vi "Scrape Matplotlib Color Map Hacking.vi"() -> ()   [LabVIEW 2019]
uses:
  <vilib>/Utility/sysdir.llb/System Directory Type.ctl
panel:
  out "Colormap Map":map{string, u32[]}(c390)
  out "Colormap Names":string[](array[string])
  out "Intensity Graph 2":dbl[][](graph)
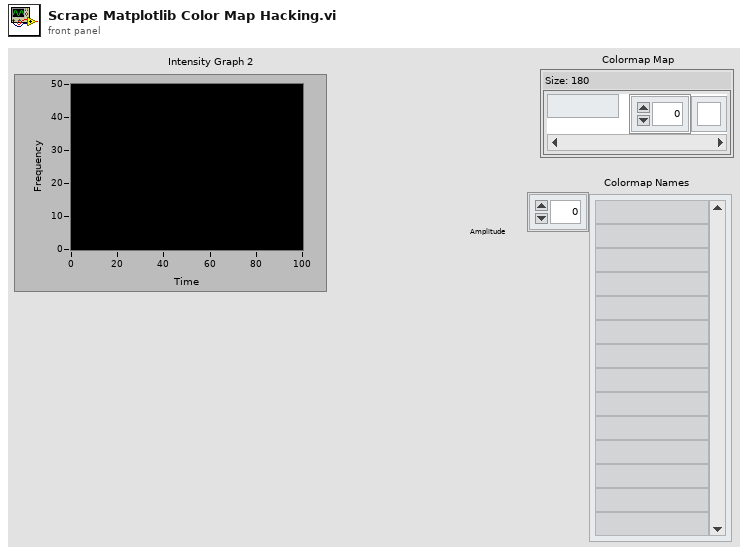
[diagram p1: front panel]
types:
  T1 = enum16{"open", "replace", "create", "open or create", "replace or create", "replace or create with confirmation"}
  T2 = typedef "System Directory Type.ctl" = i32
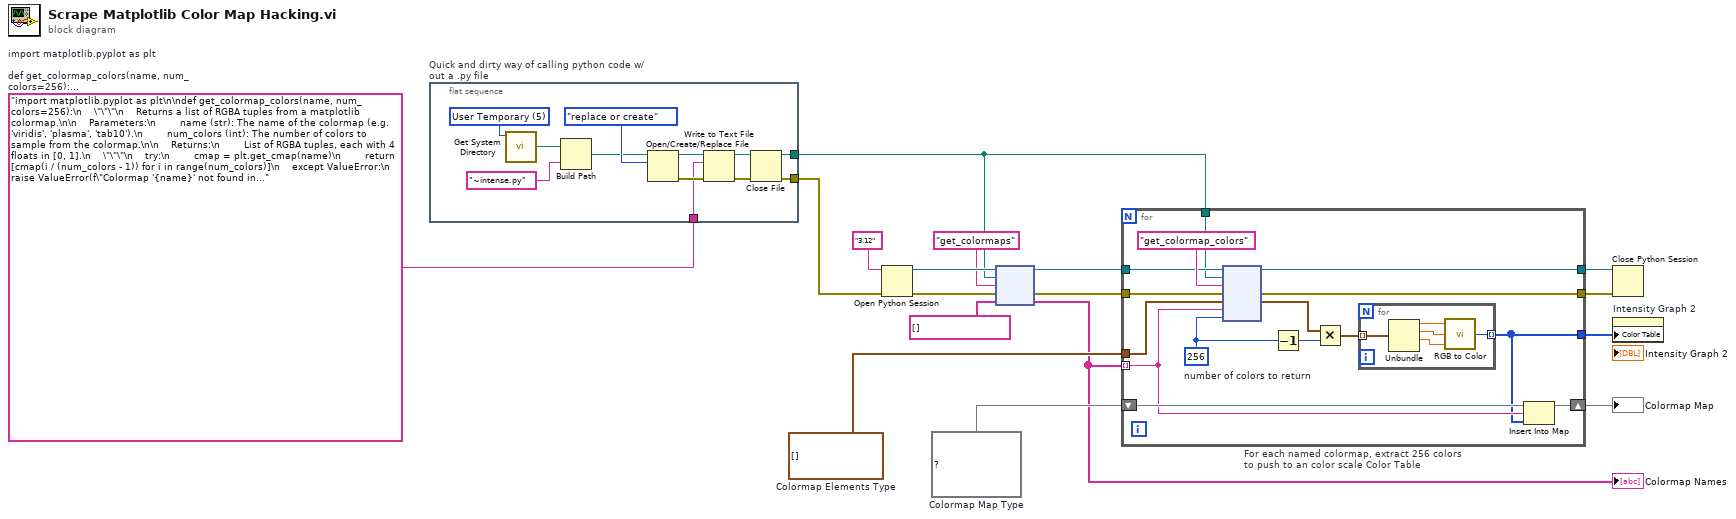
[diagram p0: block diagram]
diagram:
  w2 = cluster{"R":dbl, "G":dbl, "B":dbl, "A":dbl}[] []  # Colormap Elements Type
  w8 = map{string, u32[]} {}  # Colormap Map Type
  w3 = "import matplotlib.pyplot as plt\n\ndef get_colormap_colors(name, num_colors=256):\n    \"\"\"\n    Returns a list of RGBA tuples from a matplotlib colormap.\n\n    Parameters:\n        name (str): The name of the colormap (e.g. 'viridis', 'plasma', 'tab10').\n        num_colors (int): The number of colors to sample from the colormap.\n\n    Returns:\n        List of RGBA tuples, each with 4 floats in [0, 1].\n    \"\"\"\n    try:\n        cmap = plt.get_cmap(name)\n        return [cmap(i / (num_colors - 1)) for i in range(num_colors)]\n    except ValueError:\n        raise ValueError(f\"Colormap '{name}' not found in matplotlib.\")\n\ndef get_colormaps():\n    colormaps = plt.colormaps()\n    return colormaps\n"  # import matplotlib.pyplot as plt  def get_colormap_colors(name, num_colors=256):     """     Returns a list of RGBA tuples from a matplotlib colormap.      Parameters:         name (str): The name of the colormap (e.g. 'viridis', 'plasma', 'tab10').         num_colors (int): The number of colors to sample from the colormap.      Returns:         List of RGBA tuples, each with 4 floats in [0, 1].     """     try:         cmap = plt.get_cmap(name)         return [cmap(i / (num_colors - 1)) for i in range(num_colors)]     except ValueError:         raise ValueError(f"Colormap '{name}' not found in matplotlib.")  def get_colormaps():     colormaps = plt.colormaps()     return colormaps
  n1 = flat-sequence "Quick and dirty way of calling python code w/out a .py file" {
    tunnel: [w27] -> w16
    tunnel: [w21] -> w11
    tunnel: w3 -> [w18]
    frame #0 {
      w20 = T2 5 items=["User Home"=0, "User Desktop"=1, "User Documents"=2, "User Application Data"=3, "User Preferences"=4, "User Temporary"=5, "Public Documents"=6, "Public Application Data"=7, "Public Preferences"=8, "Public Cache"=13, "System Core Libraries"=9, "System Installed Libraries"=10, "Application Files"=11, "Boot Volume Root"=12] ("system directory type")
      n2 = call <vilib>:"Get System Directory.vi"("system directory type"=w20) -> ("system directory"=w23:path)  [unwired: 10 in]
      n3 = Build Path(base path=w23, name or relative path="~intense.py") -> (appended path=w22:path)
      n4 = Open/Create/Replace File(file path (use dialog)=w22, operation (0:open)=T1."replace or create") -> (refnum out=w26:refnum<file>, error out=w25:errorcluster)  [unwired: 4 in, 1 out]
      n5 = Write to Text File(file (use dialog)=w26, text=w18, error in=w25) -> (refnum out=w28:refnum<file>, error out=w29:errorcluster)  [unwired: 1 in, 1 out]
      n6 = Close File(refnum=w28, error in=w29) -> (path=w21:path, error out=w27:errorcluster)
    }
  }
  n7 = Open Python Session(python version="3.12" ("Python version"), 3:w16) -> (session out=w13:refnum<k35>, error out=w17:errorcluster)  [unwired: 1 in]
  n8 = node(w13, w11, "get_colormaps" ("function name"), w17, string[] [] ("function name")) -> (w12:refnum<k35>, w14:errorcluster, w1:string[])  [unwired: 2 out]
  "Colormap Names" <- w1
  n9 = for "For each named colormap, extract 256 colors to push to an color scale Color Table" {
    tunnel: [w30] -> w15
    tunnel: w14 -> [w40]
    tunnel: w12 -> [w39]
    tunnel: w11 -> [w38]
    tunnel: w1 -> [w33] mode=indexing
    shift-right: [w37] -> w5
    shift-left: w8 -> [w36]
    tunnel: [w35] -> w7
    tunnel: [w34] -> w6
    tunnel: w2 -> [w44]
    w31 = 256  # number of colors to return
    n10 = node(w39, w38, "get_colormap_colors" ("function name"), w40, w44, w33, w31) -> (w35:refnum<k35>, w34:errorcluster, w42:cluster{"R":dbl, "G":dbl, "B":dbl, "A":dbl}[])  [unwired: 2 in, 2 out]
    n11 = Decrement(x=w31) -> (x-1=w32:i32)
    n12 = Multiply(x=w42, y=w32) -> (x*y=w41:cluster{"R":dbl, "G":dbl, "B":dbl, "A":dbl}[])
    n13 = for {
      tunnel: w41 -> [w49] mode=indexing
      tunnel: [w45] -> w30 mode=indexing
      n14 = Unbundle(w49) -> ("R"=w48:dbl, "G"=w47:dbl, "B"=w46:dbl)  [unwired: 1 out]
      n15 = call <vilib>:"RGB to Color.vi"("B"=w46, "G"=w47, "R"=w48) -> ("Color"=w45:u32)
    }
    n16 = Insert Into Map(map in=w36, key=w33, value=w30) -> (map out=w37:map{string, u32[]})  [unwired: 2 out]
  }
  "Colormap Map" <- w5
  n17 = Close Python Session(session in=w7, error in=w6) -> ()  [unwired: 1 out]
  n18 = property on="Intensity Graph 2" class="IntGraph (strict)"("Color Table"=w15) -> ()  [unwired: 2 in, 2 out]
